vi "Decode &wsadata.vi"(11 "&wsdata":u8[](array[numeric]) format="%02x") -> (0 "iMaxUdpDg":u16, 1 "iMaxSockets":u16, 2 "szSystemStatus":string, 3 "szDescription":string, 5 "wHighVersion":dbl, 7 "wVersion":dbl)   [LabVIEW 2018]
panel:
  # "WSADATA\nThe WSADATA structure contains information about the Windows Sockets implementation.\n\ntypedef struct WSAData {  \nWORD wVersion;  \nWORD wHighVersion;  \nchar szDescription[WSADESCRIPTION_LEN+1];  \nchar szSystemStatus[WSASYS_STATUS_LEN+1];  \nunsigned short iMaxSockets;  \nunsigned short iMaxUdpDg;  \nchar FAR* lpVendorInfo;\n} WSADATA, *LPWSADATA;\n\nMembers\nwVersion - Version of the Windows Sockets specification that the \n   Ws2_32.dll expects the caller to use. \n\nwHighVersion - Highest version of the Windows Sockets specification \n   that this .dll can support (also encoded as above). Normally this is the same as wVersion. \n\nszDescription - Null-terminated ASCII string into which the Ws2_32.dll \n   copies a description of the Windows Sockets implementation. The \n   text (up to 256 characters in length) can contain any characters \n   except control and formatting characters: the most likely use that \n   an application can put this to is to display it (possibly truncated) in \n   a status message. \n\nszSystemStatus - Null-terminated ASCII string into which the WSs2_32.dll \n   copies relevant status or configuration information. The Ws2_32.dll \n   should use this parameter only if the information might be useful to the\n   user or support staff: it should not be considered as an extension of the \n   szDescription parameter. \n\niMaxSockets - Retained for backward compatibility, but should be ignored \n   for Windows Sockets version 2 and later, as no single value can be \n   appropriate for all underlying service providers. \n\niMaxUdpDg - Ignored for Windows Sockets version 2 and onward. The \n   iMaxUdpDg member is retained for compatibility with Windows Sockets \n   specification 1.1, but should not be used when developing new applications.\n   For the actual maximum message size specific to a particular Windows \n   Sockets service provider and socket type, applications should use \n   getsockopt to retrieve the value of option SO_MAX_MSG_SIZE after a \n   socket has been created. \n\nlpVendorInfo - Ignored for Windows Sockets version 2 and onward. It is \n   retained for compatibility with Windows Sockets specification 1.1. \n   Applications needing to access vendor-specific configuration information\n   should use getsockopt to retrieve the value of option PVD_CONFIG. The \n   definition of this value (if utilized) is beyond the scope of this specification. \n\nNote  An application should ignore the iMaxsockets, iMaxUdpDg, and lpVendorInfo \nmembers in WSADATA if the value in wVersion after a successful call to WSAStartup \nis at least 2. This is because the architecture of Windows Sockets has been \nchanged in version 2 to support multiple providers, and WSADATA no longer applies \nto a single vendor's stack. Two new socket options are introduced to supply\n provider-specific information: SO_MAX_MSG_SIZE (replaces the iMaxUdpDg element) \nand PVD_CONFIG (allows any other provider-specific configuration to occur)."
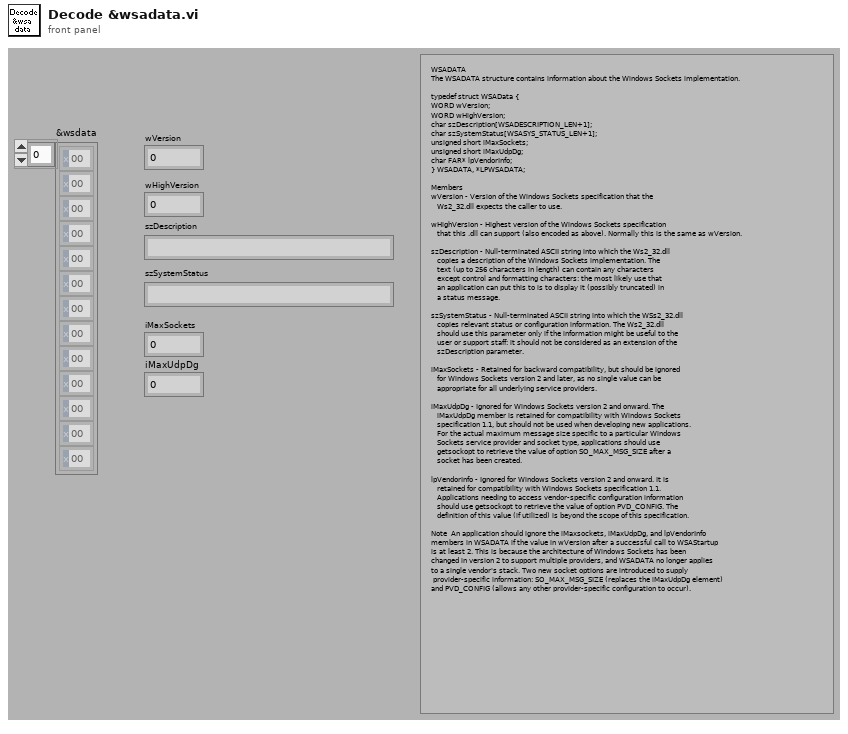
[diagram p1: front panel]
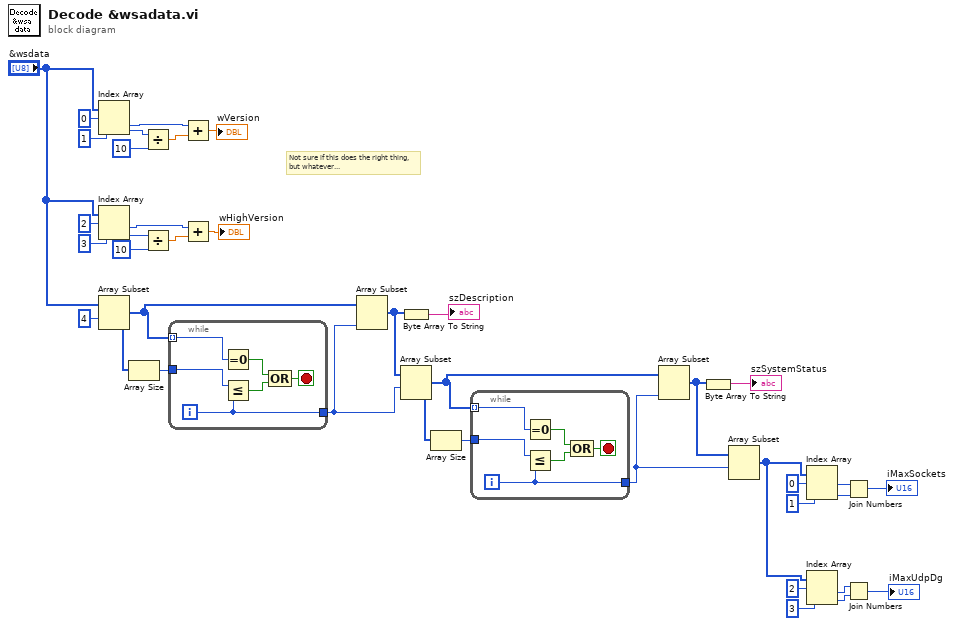
[diagram p0: block diagram]
diagram:
  # "Not sure if this does the right thing,\nbut whatever..."
  n1 = Index Array(array="&wsdata", index #1=0 ("index"), index #2=1 ("index")) -> (element #1=w26:u8, element #2=w29:u8)
  n2 = Index Array(array="&wsdata", index #1=2 ("index"), index #2=3 ("index")) -> (element #1=w21:u8, element #2=w22:u8)
  n3 = Array Subset "Array Subset"(array="&wsdata", index=4) -> (w31:u8[])  [unwired: 1 in]
  n4 = Array Size(array=w31) -> (size(s)=w32:i32)
  n5 = Divide(x=w29, y=u8 10) -> (x/y=w25:dbl)
  n6 = Divide(x=w22, y=u8 10) -> (x/y=w24:dbl)
  n7 = while {
    tunnel: w31 -> [w42] mode=indexing
    tunnel: w32 -> [w43]
    tunnel: [w38] -> w14
    i -> [w38]
    stop <- w39 stop-if-true
    n8 = Equal To 0?(x=w42) -> (x = 0?=w40:bool)
    n9 = Less Or Equal?(x=w43, y=w38) -> (x <= y?=w41:bool)
    n10 = Compound Arithmetic op=OR(w40, w41) -> (w39:bool)
  }
  n11 = Add(x=w26, y=w25) -> (x+y=→"wVersion":dbl)
  n12 = Add(x=w21, y=w24) -> (x+y=→"wHighVersion":dbl)
  n13 = Array Subset(array=w31, length=w14) -> (w15:u8[])  [unwired: 1 in]
  n14 = Byte Array To String(unsigned byte array=w15) -> (string=→"szDescription":string)
  n15 = Array Subset "Array Subset"(array=w15, index=w14) -> (w19:u8[])  [unwired: 1 in]
  n16 = Array Size(array=w19) -> (size(s)=w18:i32)
  n17 = while {
    tunnel: w19 -> [w48] mode=indexing
    tunnel: w18 -> [w49]
    tunnel: [w44] -> w8
    i -> [w44]
    stop <- w45 stop-if-true
    n18 = Equal To 0?(x=w48) -> (x = 0?=w46:bool)
    n19 = Less Or Equal?(x=w49, y=w44) -> (x <= y?=w47:bool)
    n20 = Compound Arithmetic op=OR(w46, w47) -> (w45:bool)
  }
  n21 = Array Subset(array=w19, length=w8) -> (w9:u8[])  [unwired: 1 in]
  n22 = Byte Array To String(unsigned byte array=w9) -> (string=→"szSystemStatus":string)
  n23 = Array Subset "Array Subset"(array=w9, index=w8) -> (w7:u8[])  [unwired: 1 in]
  n24 = Index Array(array=w7, index #1=0 ("index"), index #2=1 ("index")) -> (element #1=w5:u8, element #2=w6:u8)
  n25 = Index Array(array=w7, index #1=2 ("index"), index #2=3 ("index")) -> (element #1=w3:u8, element #2=w2:u8)
  n26 = Join Numbers(hi=w5, lo=w6) -> ((hi.lo)=→"iMaxSockets":u16)
  n27 = Join Numbers(hi=w3, lo=w2) -> ((hi.lo)=→"iMaxUdpDg":u16)
